vi "ini_sesion.vi"(8 "error in (no error)":errorcluster, 11 "5785_3.2GHz_one channel in":refnum<class "5785_3.2GHz_one channel.lvclass">) -> (0 "error out":errorcluster, 3 "5785_3.2GHz_one channel out":refnum<class "5785_3.2GHz_one channel.lvclass">)   [LabVIEW 2021, in "5785_3.2GHz_one channel.lvclass"]
uses:
  5785_3.2GHz_one channel.lvclass
  5785_3.2GHz_one channel.lvclass/5785_3.2GHz_one channel.ctl
  <instrlib>/FlexRIO/API/Host/v1/NI FlexRIO/API/Reference Clock Source.ctl
  <instrlib>/FlexRIO/API/Host/v1/NI FlexRIO API v1.lvlib
  <resource>/objmgr/niflexrioapiStream.rc
  <resource>/objmgr/niflexrioapi.rc
  <vilib>/rvi/interface/nirviOpenFPGA/nirviOpenFPGA.xnode
  FPGA Bitfiles/pulsetx_PXIe-5785(KU060)_3GHz_IBW.lvbitx
  <vilib>/rvi/interface/nirviMethod/nirviMethod.xnode
  <vilib>/FPGAPlugInAG/Dynamic/niLvFpga_ConfigureFifo_Dynamic.vi
  <vilib>/rvi/errors/niLvFpgaMergeErrorWithErrorCode.vi
  <resource>/objmgr/niflexrioapiChannel.rc
  <vilib>/rvi/interface/nirviReadWriteControl/nirviReadWriteControl.xnode
  NiFpgaLv.dll
  <vilib>/Utility/error.llb/Error Cluster From Error Code.vi
  <vilib>/rvi/interface/Simulation/niFpgaSimulationCallBeginRW.vi
  <vilib>/rvi/errors/niLvFpgaAdjustHostInterfaceError.vi
  <vilib>/FPGAPlugInAG/Dynamic/niLvFpga_StopFifo_Dynamic.vi
  <instrlib>/FlexRIO/API/Host/v1/NI FlexRIO/API/Configure Reference Clock.vi
  <instrlib>/FlexRIO/API/Host/v1/NI FlexRIO/API/Get Property Reference - Fpga Small.vi
  <vilib>/FPGAPlugInAG/PXIe-5785 (KU060)/niLvFpga_Open_PXIe-5785 (KU060).vi
  <vilib>/rvi/interface/common/dynamic/niFpgaDynamicAddResources.vi
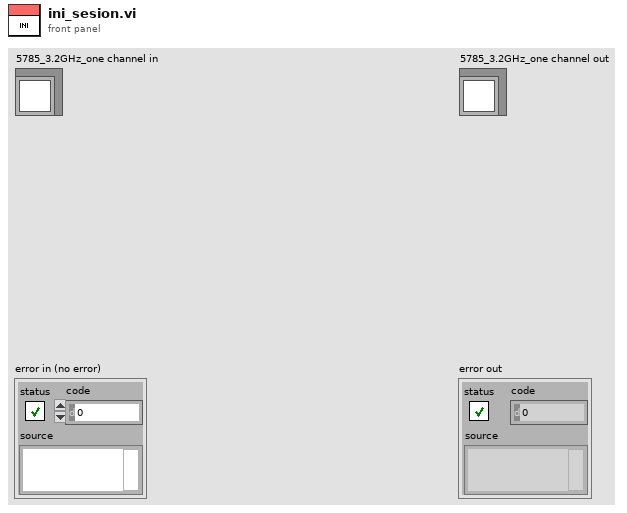
[diagram p1: front panel]
types:
  T1 = typedef "nirio_resource_hc.ctl" = tag
  T2 = typedef "NI FlexRIO API v1.lvlib/Reference Clock Source.ctl" = i32
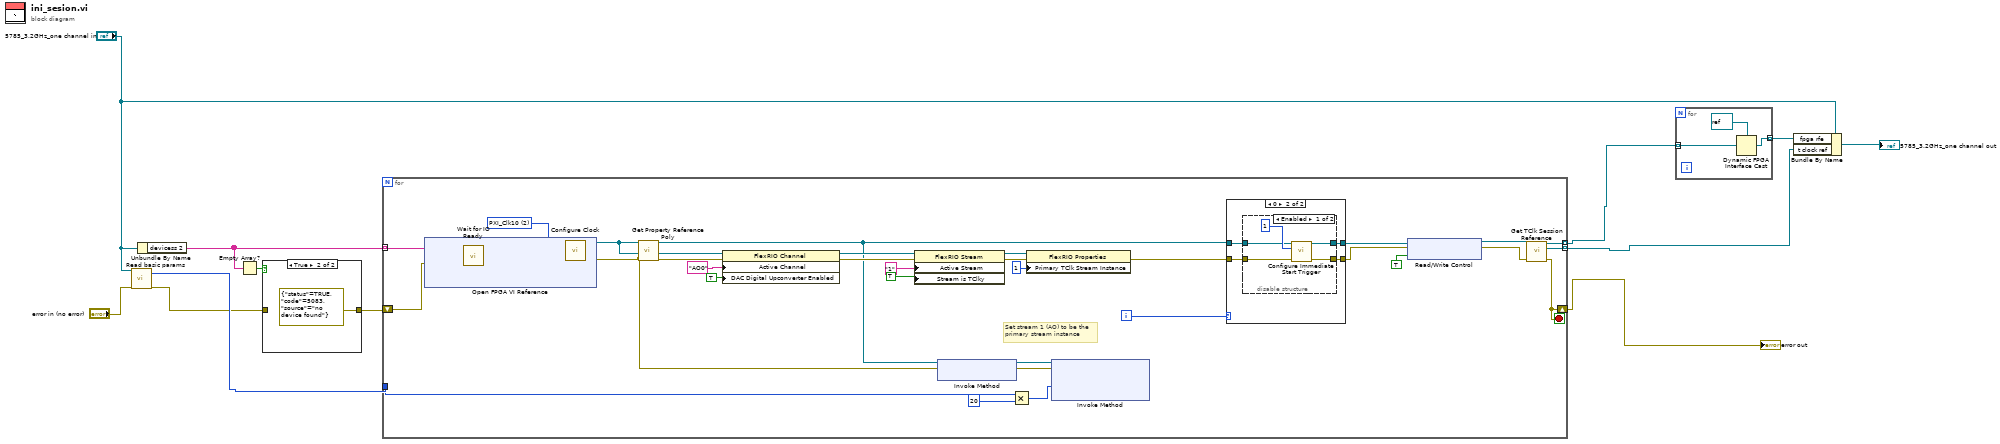
[diagram p0: block diagram]
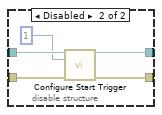
[diagram p4: hidden frame]
diagram:
  n1 = call-dynamic "Read basic params.vi"("device_type in"="5785_3.2GHz_one channel in", "error in (no error)"="error in (no error)") -> ("buffer size"=w3:u32, "error out"=w1:errorcluster)  [unwired: 12 in, 4 out]
  n2 = Unbundle By Name("5785_3.2GHz_one channel in") -> ("devicess 2"=w9:T1[])
  n3 = Empty Array?(array=w9) -> (empty?=w8:bool)
  n4 = case shown="True" w8 {
    tunnel: [w13 errorcluster {"status"=TRUE, "code"=5083, "source"="no device found"} ("error in (no error)")] -> w7
    tunnel: w1 -> [w13 _]
    frame False {
    }
    frame True {
    }
  }
  n5 = for {
    tunnel: [w44] -> w11 mode=indexing
    shift-right: [w25] -> w6
    shift-left: w7 -> [w38]
    tunnel: [w43] -> w12 mode=indexing
    tunnel: w3 -> [w37]
    tunnel: w9 -> [w29] mode=indexing
    i -> [w41]
    stop <- w25 stop-if-true
    w28 = T2 2 items=["Default", "Onboard", "PXI_Clk10", "External", "None", "Baseboard Reference"] ("reference clock source")
    # "Set stream 1 (AO) to be the\nprimary stream instance"
    n6 = xnode "Open FPGA VI Reference"("error in"=w38, "resource name"=w29) -> ("FPGA VI Reference Out"=w40:refnum<k20>, "error out"=w39:errorcluster)
    n7 = call <instrlib>:"Wait for IO Ready.vi"("fpga interface in"=w40, "error in"=w39) -> ("fpga interface out"=w27:refnum<k20>, "error out"=w26:errorcluster)  [unwired: 10 in, 2 out]
    n8 = call-poly <instrlib>:"Configure Clock.vi"("fpga interface in"=w27, "reference clock source"=w28, "error in"=w26) -> ("fpga interface out"=w19:refnum<k20>, "error out"=w18:errorcluster)  [unwired: 11 in]
    n9 = call-poly <instrlib>:"Get Property Reference Poly.vi"("error in (no error)"=w18, "fpga interface in"=w19) -> ("error out"=w32:errorcluster, "property reference"=w33:refnum<k20>)  [unwired: 4 in, 1 out]
    n10 = property class="FlexRIO Channel"(reference=w33, error in=w32, "Active Channel"="AO0", "DAC Digital Upconverter Enabled"=TRUE ("Analog Output:DAC Digital Upconverter Enabled")) -> (reference out=w31:refnum<k20>, error out=w30:errorcluster)
    n11 = property class="FlexRIO Stream"(reference=w31, error in=w30, "Active Stream"="1", "Stream is TClky"=TRUE ("Configuration:Stream is TClky")) -> (reference out=w47:refnum<k20>, error out=w46:errorcluster)
    n12 = xnode "Invoke Method"("FPGA VI Reference In"=w19, "error in"=w18) -> ("FPGA VI Reference Out"=w16:refnum<k20>, "error out"=w17:errorcluster)
    n13 = Multiply(x=w37, y=u32 20) -> (x*y=w36:u32)
    n14 = property class="FlexRIO Properties"(reference=w47, error in=w46, "Primary TClk Stream Instance"=1 ("Device:Primary TClk Stream Instance")) -> (error out=w42:errorcluster)  [unwired: 1 out]
    n15 = xnode "Invoke Method"("FPGA VI Reference In"=w16, "error in"=w17, "Requested Depth"=w36) -> ()  [unwired: 3 out]
    n16 = case shown="0" w41 {
      tunnel: w19 -> [w51 w55]
      tunnel: [w51 w54] -> w24
      tunnel: [w50 w53] -> w21
      tunnel: w42 -> [w50 w52]
      frame 1, Default {
      }
      frame 0 {
        n17 = disable-structure shown="Enabled" {
          disable-tunnel: w55 -> [w59 w65]
          disable-tunnel: [w58 w63] -> w54
          disable-tunnel: [w57 w62] -> w53
          disable-tunnel: w52 -> [w56 w61]
          frame Enabled {
            n18 = call <instrlib>:"Configure Immediate Start Trigger.vi"("fpga interface in"=w59, "trigger instance"=u32 1, "error in"=w56) -> ("fpga interface out"=w58:refnum<k20>, "error out"=w57:errorcluster)  [unwired: 10 in, 1 out]
          }
          frame Disabled {
            n19 = call-poly <instrlib>:"Configure Start Trigger.vi"("fpga interface in"=w65, "trigger instance"=u32 1, "error in"=w61) -> ("fpga interface out"=w63:refnum<k20>, "error out"=w62:errorcluster)  [unwired: 10 in, 1 out]
          }
        }
      }
    }
    n20 = xnode "Read/Write Control"("FPGA VI Reference In"=w24, "error in"=w21, "reset system clock"=TRUE) -> ("FPGA VI Reference Out"=w23:refnum<k20>, "error out"=w22:errorcluster)
    n21 = call <instrlib>:"Get TClk Session Reference.vi"("fpga interface in"=w23, "error in"=w22) -> ("fpga interface out"=w44:refnum<k20>, "tclk session reference"=w43:refnum<k20>, "error out"=w25:errorcluster)  [unwired: 11 in]
  }
  "error out" <- w6
  n22 = for {
    tunnel: w11 -> [w67] mode=indexing
    tunnel: [w66] -> w10 mode=indexing
    n23 = Dynamic FPGA Interface Cast(Session In=refnum<k20> refnum ("fpga interface out"), Type=w67) -> (Session Out=w66:refnum<k20>)
  }
  n24 = Bundle By Name(cluster="5785_3.2GHz_one channel in", "fpga rfe"=w10, "t clock ref"=w12) -> (→"5785_3.2GHz_one channel out":refnum<class "5785_3.2GHz_one channel.lvclass">)
